vi "ballScrewControl.vi"(0 "joy1Wheel":dbl, 1 "button8":bool, 4 "button7":bool, 5 "ballScrewMotorIN":T1={"DeviceStatus"={"status"=FALSE, "code"=0, "source"=""}, "Type"=enum."PWM", "PWM"={"Digital Module"=enum."Digital Module 2", "PWM Channel"=enum."PWM 1", "DeadBand"={"Name"="", "maxPositivePwm"=0, "minPositivePwm"=0, "centerPwm"=0, "maxNegativePwm"=0, "minNegativePwm"=0, "angularRange"=0}}, "CAN"={"Device Number"=0, "Control Mode"=enum."Percent VBus", "Semaphore"=refnum, "Max Vout"=12.0}, "Invert"=FALSE, "TransformRef"=refnum, "InvTransformRef"=refnum}, 6 "Distance":dbl, 7 "joy2YAxis":dbl, 8 "autoTrackingButton":bool, 9 "closedLoopKillButton":bool, 10 "ballScrewBotLimitSwitch":bool, 11 "ballScrewTopLimitSwitch":bool) -> (2 "motorValueOutput":dbl, 3 "ballScrewMotorOUT":T1={"DeviceStatus"={"status"=FALSE, "code"=0, "source"=""}, "Type"=enum."PWM", "PWM"={"Digital Module"=enum."Digital Module 1", "PWM Channel"=enum."Invalid", "DeadBand"={"Name"="", "maxPositivePwm"=0, "minPositivePwm"=0, "centerPwm"=0, "maxNegativePwm"=0, "minNegativePwm"=0, "angularRange"=0}}, "CAN"={"Device Number"=0, "Control Mode"=enum."Percent VBus", "Semaphore"=refnum, "Max Vout"=12.0}, "Invert"=FALSE, "TransformRef"=refnum, "InvTransformRef"=refnum})   [LabVIEW 2012]
uses:
  <vilib>/Rock Robotics/WPI/MotorControl/WPI_MotorControlDeviceRef.ctl
  <vilib>/Rock Robotics/SystemInterfaces/Typedef/FPGA_TypedefDigitalModule.ctl
  <vilib>/Rock Robotics/SystemInterfaces/DIO/FPGA_DIOPWMChannel.ctl
  <vilib>/Rock Robotics/WPI/PWM/WPI_PWMDeadband.ctl
  <vilib>/Rock Robotics/WPI/CAN/Jaguar/SubVIs/WPI_CANJaguar_ControlMode.ctl
  <vilib>/Rock Robotics/WPI/PWM/WPI_PWMTransform_ConPane.ctl
  <vilib>/Rock Robotics/WPI/CAN/Jaguar/SubVIs/WPI_CANJaguar_StatusSelect.ctl
  <vilib>/Rock Robotics/WPI/CAN/Jaguar/SubVIs/WPI_CANJaguar_StatusChannelSelect.ctl
  <vilib>/Rock Robotics/WPI/DriverStation/DriverStationLCD/WPI_DriverStationLCDLCDLine.ctl
  <vilib>/Rock Robotics/WPI/CAN/Jaguar/SubVIs/WPI_CANJaguar_BrakeCoastMode.ctl
  2013NewCan/Robot Global Data.vi
panel:
  out "POT FEEDBACK":dbl
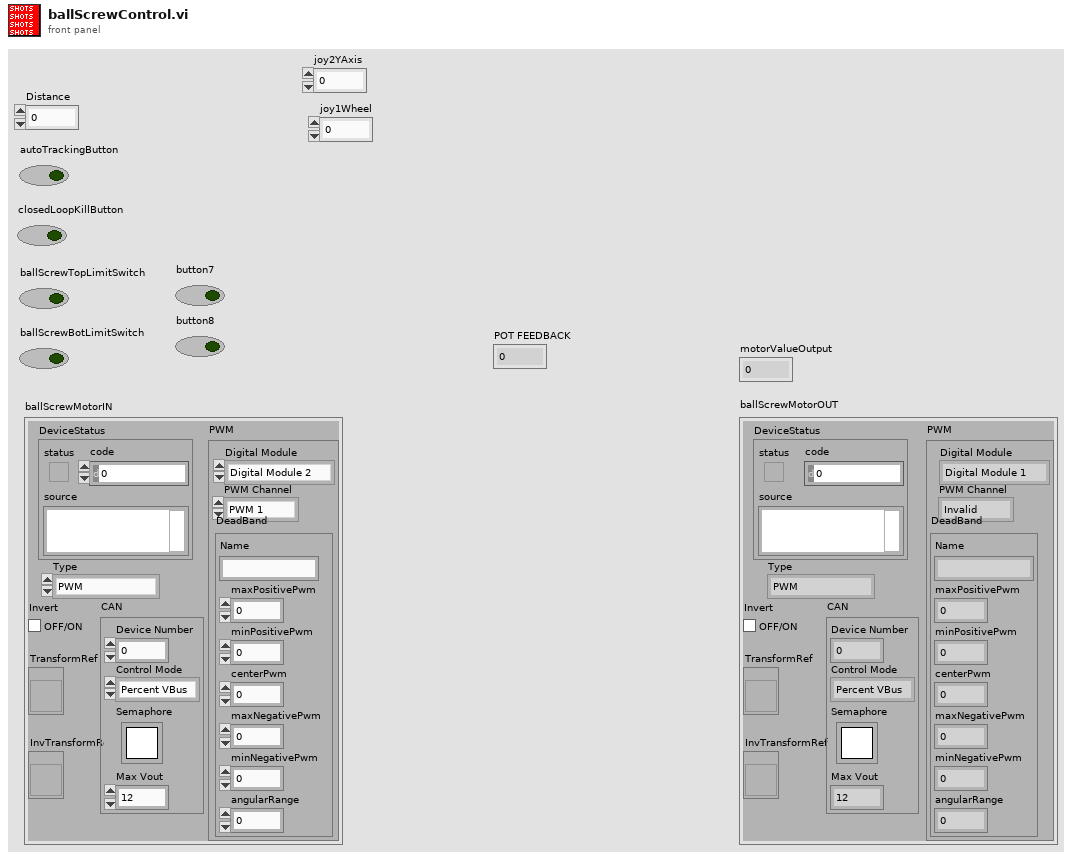
[diagram p1: front panel]
types:
  T1 = typedef "WPI_MotorControlDeviceRef.ctl" = cluster{"DeviceStatus":errorcluster, "Type":enum16{"PWM", "CAN"}, "PWM":cluster{"Digital Module":T2, "PWM Channel":T3, "DeadBand":T4}, "CAN":cluster{"Device Number":u8, "Control Mode":T5, "Semaphore":T6, "Max Vout":dbl}, "Invert":bool, "TransformRef":T7, "InvTransformRef":T7}
  T2 = typedef "FPGA_TypedefDigitalModule.ctl" = enum16{"Digital Module 1", "Digital Module 2"}
  T3 = typedef "FPGA_DIOPWMChannel.ctl" = enum8{"PWM 1", "PWM 2", "PWM 3", "PWM 4", "PWM 5", "PWM 6", "PWM 7", "PWM 8", "PWM 9", "PWM 10", "Invalid"}
  T4 = typedef "WPI_PWMDeadband.ctl" = cluster{"Name":string, "maxPositivePwm":i32, "minPositivePwm":i32, "centerPwm":i32, "maxNegativePwm":i32, "minNegativePwm":i32, "angularRange":u16}
  T5 = typedef "WPI_CANJaguar_ControlMode.ctl" = enum8{"Percent VBus", "Current", "Speed", "Position", "Voltage"}
  T6 = typedef "Semaphore RefNum" = refnum<k1>
  T7 = typedef "WPI_PWMTransform_ConPane.ctl" = refnum<vi>
  T8 = typedef "WPI_DriverStationLCDLCDLine.ctl" = enum16{"Main - Line 1", "User - Line 2", "User - Line 3", "User - Line 4", "User - Line 5", "User - Line 6"}
  T9 = typedef "WPI_CANJaguar_StatusChannelSelect.ctl" = enum16{"Periodic Status Channel 1", "Periodic Status Channel 2", "Periodic Status Channel 3", "Periodic Status Channel 4", "On Demand Status"}
  T10 = typedef "WPI_CANJaguar_StatusSelect.ctl" = enum16{"Output Percent VBus", "Output Voltage", "Bus Voltage", "Current", "Temperature", "Position", "Speed", "Limit Switches", "Faults", "Fault Counters", "Power Cycle"}
  T11 = typedef "WPI_CANJaguar_Status.ctl" = cluster{"Output Percent VBus":dbl, "Output Voltage":dbl, "Bus Voltage":dbl, "Current":dbl, "Temperature":dbl, "Position":dbl, "Speed":dbl, "Limits":cluster{"Forward Limit":bool, "Reverse Limit":bool, "Forward Soft Limit":bool, "Reverse Soft Limit":bool, "Sticky Forward Limit":bool, "Sticky Reverse Limit":bool, "Sticky Forward Soft Limit":bool, "Sticky Reverse Soft Limit":bool}, "Faults":cluster{"Current Fault":bool, "Temperature Fault":bool, "Bus Voltage Fault":bool, "Gate Driver Fault":bool, "Comm Fault":bool}, "Fault Counters":cluster{"Current Faults":u8, "Temperature Faults":u8, "Bus Voltage Faults":u8, "Gate Driver Faults":u8, "Comm Faults":u8, "CAN Status":u8, "CAN RX Errors":u8, "CAN TX Errors":u8}, "Power Cycle":bool}
  T12 = typedef "WPI_CANJaguar_BrakeCoastMode.ctl" = enum8{"Jumper", "Brake", "Coast"}
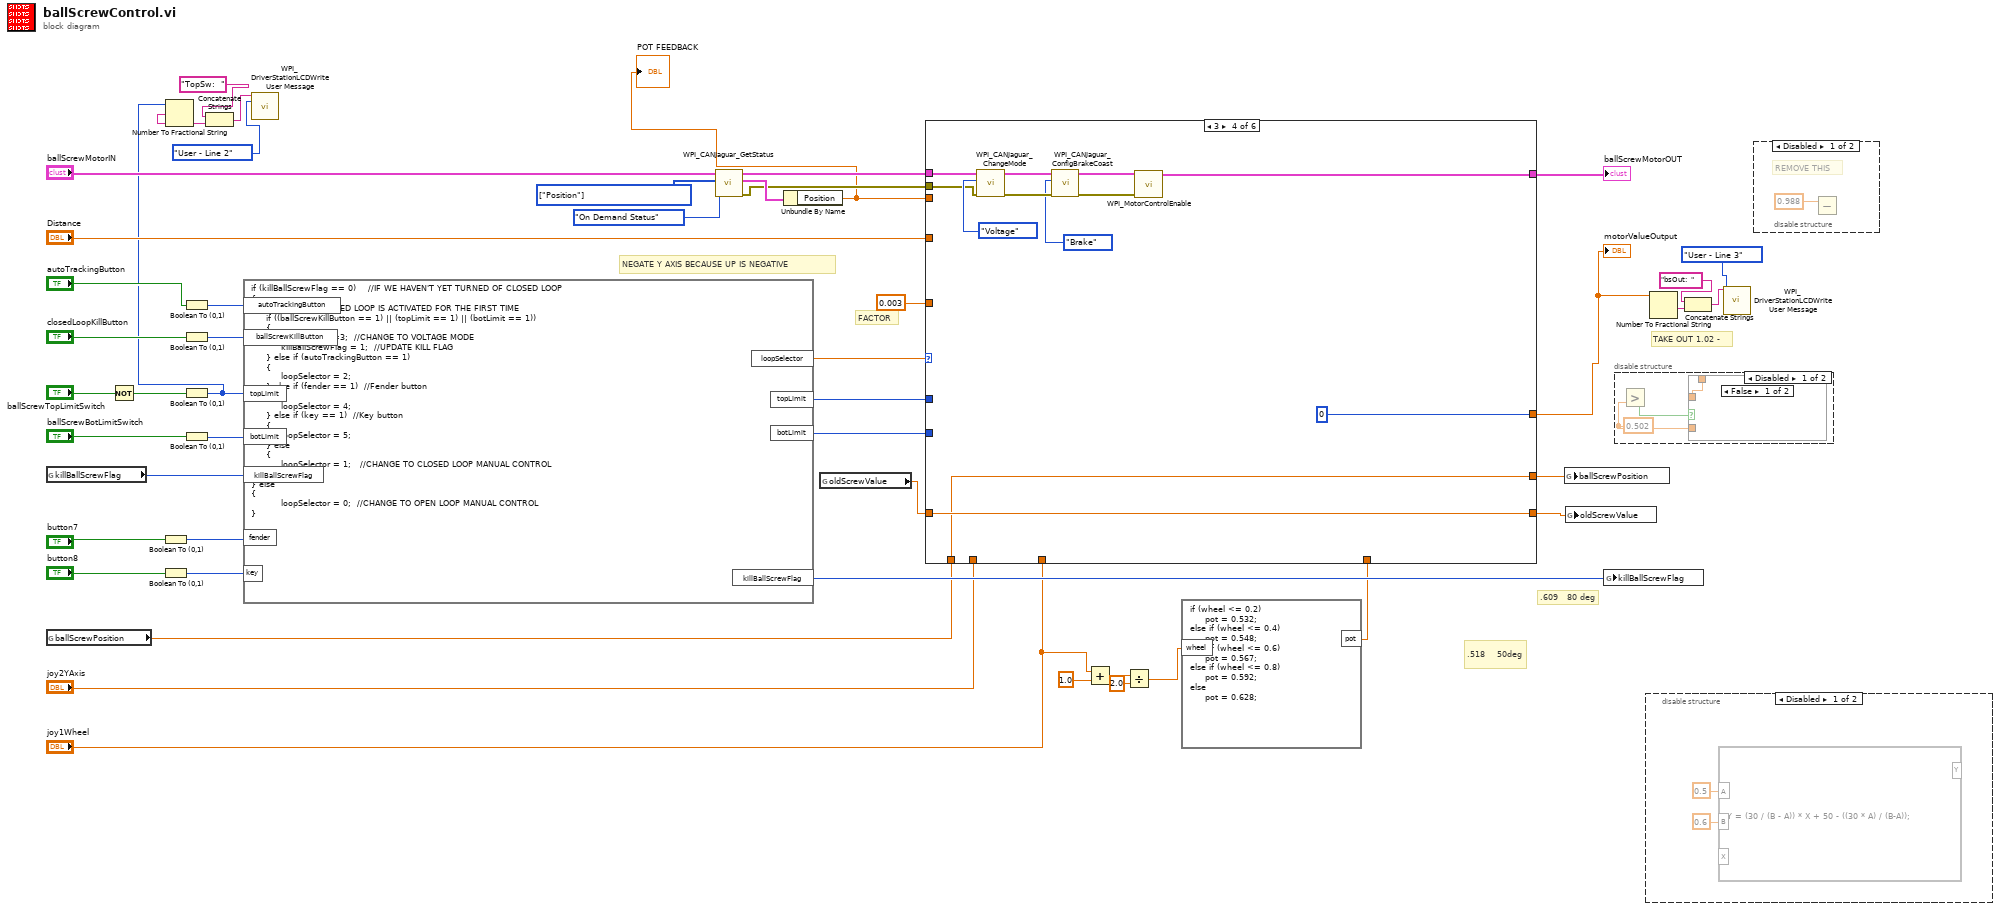
[diagram p0: block diagram]
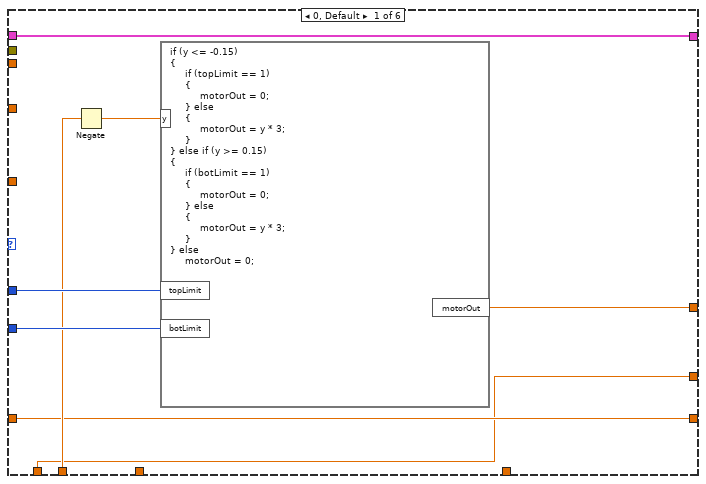
[diagram p6: hidden frame]
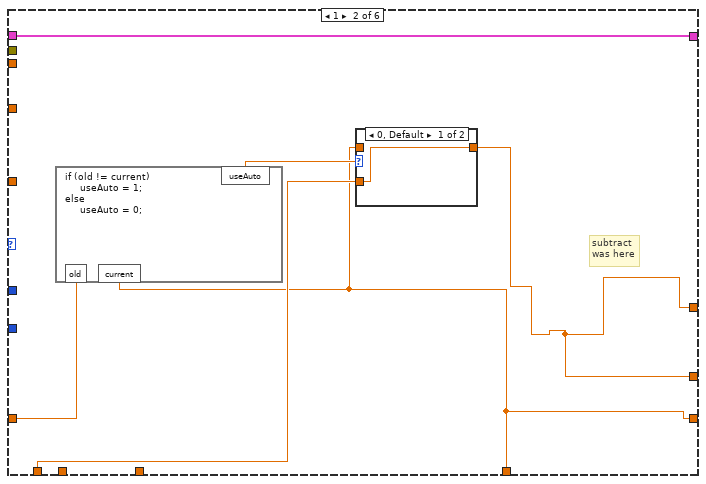
[diagram p7: hidden frame]
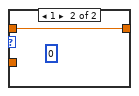
[diagram p8: hidden frame]
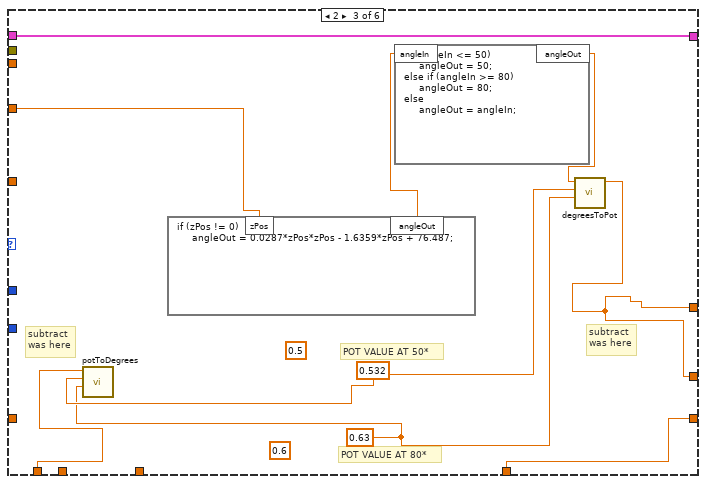
[diagram p9: hidden frame]
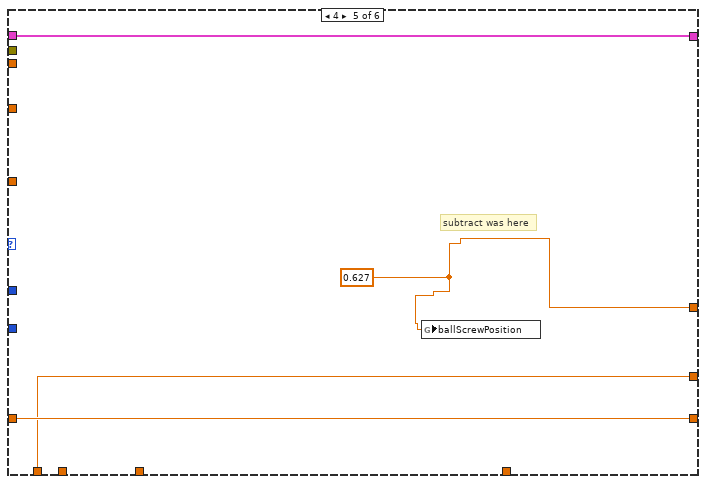
[diagram p10: hidden frame]
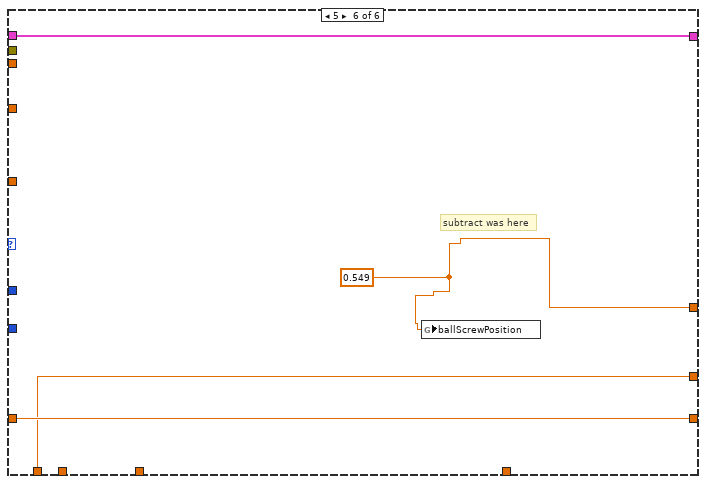
[diagram p11: hidden frame]
diagram:
  w30 = T10[] [enum."Position"] items=["Output Percent VBus", "Output Voltage", "Bus Voltage", "Current", "Temperature", "Position", "Speed", "Limit Switches", "Faults", "Fault Counters", "Power Cycle"] ("Status Select")
  # ".609   80 deg"
  # ".518    50deg"
  # "TAKE OUT 1.02 -"
  # "FACTOR"
  # "NEGATE Y AXIS BECAUSE UP IS NEGATIVE"
  n1 = global read "Robot Global Data.vi" "killBallScrewFlag"() -> (w47:i8)
  n2 = global read "Robot Global Data.vi" "ballScrewPosition"() -> (w34:dbl)
  n3 = Not(x="ballScrewTopLimitSwitch") -> (.not. x?=w32:bool)
  n4 = Boolean To (0,1)(Boolean="button7") -> (0, 1=w18:i16)
  n5 = Boolean To (0,1)(Boolean="button8") -> (0, 1=w2:i16)
  n6 = Boolean To (0,1)(Boolean="autoTrackingButton") -> (0, 1=w36:i16)
  n7 = Boolean To (0,1)(Boolean="closedLoopKillButton") -> (0, 1=w48:i16)
  n8 = Boolean To (0,1)(Boolean=w32) -> (0, 1=w19:i16)
  n9 = Number To Fractional String(number=w19) -> (F-format string=w23:string)  [unwired: 3 in]
  n10 = Boolean To (0,1)(Boolean="ballScrewBotLimitSwitch") -> (0, 1=w24:i16)
  n11 = Concatenate Strings("TopSw:  " ("line text"), w23) -> (w22:string)
  n12 = formula code="if (killBallScrewFlag == 0)    //IF WE HAVEN'T YET TURNED OF CLOSED LOOP\n{\n     //IF THE KILL CLOSED LOOP IS ACTIVATED FOR THE FIRST TIME\n     if ((ballScrewKillButton == 1) || (topLimit == 1) || (botLimit == 1))\n     {\n          loopSelector =3;  //CHANGE TO VOLTAGE MODE\n          killBallScrewFlag = 1;  //UPDATE KILL FLAG\n     } else if (autoTrackingButton == 1)\n     {\n          loopSelector = 2;\n     } else if (fender == 1)  //Fender button\n     {\n          loopSelector = 4;\n     } else if (key == 1)  //Key button\n     {\n          loopSelector = 5;\n     } else\n     {\n          loopSelector = 1;   //CHANGE TO CLOSED LOOP MANUAL CONTROL\n     }\n} else\n{\n          loopSelector = 0;  //CHANGE TO OPEN LOOP MANUAL CONTROL\n}"("ballScrewKillButton"=w48, "killBallScrewFlag"=w47, "botLimit"=w24, "topLimit"=w19, "autoTrackingButton"=w36, "fender"=w18, "key"=w2) -> ("loopSelector"=w25:dbl, "killBallScrewFlag"=w43:i8, "topLimit"=w38:i16, "botLimit"=w39:i16)
  n13 = call <vilib>:"WPI_DriverStationLCDWrite User Message.vi"("line text"=w22, "line"=WPI_DriverStationLCDLCDLine."User - Line 2") -> ()  [unwired: 13 in, 1 out]
  n14 = call <vilib>:"WPI_CANJaguar_GetStatus.vi"("Status Channel Select"=WPI_CANJaguar_StatusChannelSelect."On Demand Status", "Status Select"=w30, "CAN Jaguar Ref"="ballScrewMotorIN") -> ("error out"=w31:errorcluster, "Status"=w40:T11, "CAN Jaguar Ref Out"=w41:T1)  [unwired: 6 in]
  n15 = Unbundle By Name(w40) -> ("Position"=w28:dbl)
  "POT FEEDBACK" <- w28
  n16 = global read "Robot Global Data.vi" "oldScrewValue"() -> (w9:dbl)
  n17 = Add(x="joy1Wheel", y=1.0) -> (x+y=w15:dbl)
  n18 = Divide(x=w15, y=2.0) -> (x/y=w13:dbl)
  n19 = formula code="if (wheel <= 0.2)\n     pot = 0.532;\nelse if (wheel <= 0.4)\n     pot = 0.548;\nelse if (wheel <= 0.6)\n     pot = 0.567;\nelse if (wheel <= 0.8)\n     pot = 0.592;\nelse\n     pot = 0.628;"("wheel"=w13) -> ("pot"=w11:dbl)
  n20 = case shown="3" w25 {
    tunnel: w41 -> [w56 w62 w73 w85 w89 w93]
    tunnel: [w56 w62 w73 w84 w89 w93] -> w44
    tunnel: w28 -> [_ _ _ _ _ _]
    tunnel: w34 -> [w49 w59 w67 w74 w87 w91]
    tunnel: [w53 w57 w68 0 w86 w90] -> w3
    tunnel: w39 -> [w55 _ _ _ _ _]
    tunnel: w38 -> [w54 _ _ _ _ _]
    tunnel: 0.003 ("input variable") -> [_ _ _ _ _ _]
    tunnel: w31 -> [_ _ _ w81 _ _]
    tunnel: "Distance" -> [_ _ w70 _ _ _]
    tunnel: "joy1Wheel" -> [_ _ _ _ _ _]
    tunnel: "joy2YAxis" -> [w51 _ _ _ _ _]
    tunnel: w11 -> [_ w58 w69 _ _ _]
    tunnel: [w50 w58 w69 w75 w88 w92] -> w10
    tunnel: w9 -> [w50 w61 _ w75 w88 w92]
    tunnel: [w49 w57 w68 w74 w87 w91] -> w8
    frame 0, Default {
      n21 = Negate(x=w51) -> (-x=w52:dbl)
      n22 = formula code="if (y <= -0.15)\n{\n     if (topLimit == 1)\n     {\n          motorOut = 0;\n     } else\n     {\n          motorOut = y * 3;\n     }\n} else if (y >= 0.15)\n{\n     if (botLimit == 1)\n     {\n          motorOut = 0;\n     } else\n     {\n          motorOut = y * 3;\n     }\n} else\n     motorOut = 0;"("topLimit"=w54, "botLimit"=w55, "y"=w52) -> ("motorOut"=w53:dbl)
    }
    frame 1 {
      # "subtract\nwas here"
      n23 = formula code="if (old != current)\n     useAuto = 1;\nelse\n     useAuto = 0;"("old"=w61, "current"=w58) -> ("useAuto"=w60:dbl)
      n24 = case shown="0, Default" w60 {
        tunnel: [w63 w64] -> w57
        tunnel: w58 -> [_ w64]
        tunnel: w59 -> [w63 _]
        frame 0, Default {
        }
        frame 1 {
          (unwired) 0
        }
      }
    }
    frame 2 {
      (unwired) 0.6
      (unwired) 0.5
      w71 = 0.63
      w72 = 0.532
      # "subtract\nwas here"
      # "subtract\nwas here"
      # "POT VALUE AT 50*"
      # "POT VALUE AT 80*"
      n25 = call "potToDegrees.vi"("POT VALUE AT 80*"=w71, "POT VALUE AT 50*"=w72, "POT VALUE"=w67) -> ()  [unwired: 8 in, 1 out]
      n26 = formula code="if (zPos != 0)\n     angleOut = 0.0287*zPos*zPos - 1.6359*zPos + 76.487;"("zPos"=w70) -> ("angleOut"=w66:dbl)
      n27 = formula code="if (angleIn <= 50)\n     angleOut = 50;\nelse if (angleIn >= 80)\n     angleOut = 80;\nelse\n     angleOut = angleIn;"("angleIn"=w66) -> ("angleOut"=w65:dbl)
      n28 = call "degreesToPot.vi"("POT VALUE AT 80*"=w71, "POT VALUE AT 50*"=w72, "ANGLE(DEGREES)"=w65) -> ("POT VALUE (0-1)"=w68:dbl)  [unwired: 8 in]
    }
    frame 3 {
      n29 = call <vilib>:"WPI_CANJaguar_ChangeMode.vi"("error in (no error)"=w81, "Control Mode"=WPI_CANJaguar_ControlMode."Voltage", "CAN Jaguar Ref"=w85) -> ("error out"=w79:errorcluster, "CAN Jaguar Ref Out"=w80:T1)  [unwired: 7 in]
      n30 = call <vilib>:"WPI_CANJaguar_ConfigBrakeCoast.vi"("error in (no error)"=w79, "Brake / Coast Mode"=WPI_CANJaguar_BrakeCoastMode."Brake", "CAN Jaguar Ref"=w80) -> ("error out"=w78:errorcluster, "CAN Jaguar Ref Out"=w77:T1)  [unwired: 7 in]
      n31 = call <vilib>:"WPI_MotorControlEnable.vi"("error in (no error)"=w78, "CAN Jaguar Ref"=w77) -> ("CAN Jaguar Ref Out"=w84:T1)  [unwired: 8 in, 1 out]
    }
    frame 4 {
      w86 = 0.627 ("ballScrewPosition")
      # "subtract was here"
      n32 = global write "Robot Global Data.vi" "ballScrewPosition"(w86) -> ()
    }
    frame 5 {
      w90 = 0.549 ("ballScrewPosition")
      # "subtract was here"
      n33 = global write "Robot Global Data.vi" "ballScrewPosition"(w90) -> ()
    }
  }
  "ballScrewMotorOUT" <- w44
  "motorValueOutput" <- w3
  n34 = global write "Robot Global Data.vi" "ballScrewPosition"(w8) -> ()
  n35 = global write "Robot Global Data.vi" "oldScrewValue"(w10) -> ()
  n36 = global write "Robot Global Data.vi" "killBallScrewFlag"(w43) -> ()
  n37 = disable-structure shown="Disabled" {
    frame Disabled {
      w94 = 0.502 ("y")
      n38 = Greater?(y=w94) -> (0:w95:bool)  [unwired: 1 in]
      n39 = case shown="False" w95 {
        tunnel: [w96 w97] -> _
        tunnel: _ -> [w96 _]
        tunnel: w94 -> [_ w97]
        frame False {
        }
        frame True {
        }
      }
    }
    frame Enabled {
    }
  }
  n40 = disable-structure shown="Disabled" {
    frame Disabled {
      n41 = formula code="Y = (30 / (B - A)) * X + 50 - ((30 * A) / (B-A));"("B"=0.6 ("input variable"), "A"=0.5 ("input variable")) -> ("X"=w98:dbl)  [unwired: 1 out]
    }
    frame Enabled {
    }
  }
  n42 = Number To Fractional String(number=w3) -> (F-format string=w4:string)  [unwired: 3 in]
  n43 = Concatenate Strings("bsOut:  " ("line text"), w4) -> (w5:string)
  n44 = call <vilib>:"WPI_DriverStationLCDWrite User Message.vi"("line text"=w5, "line"=WPI_DriverStationLCDLCDLine."User - Line 3") -> ()  [unwired: 13 in, 1 out]
  n45 = disable-structure shown="Disabled" {
    frame Disabled {
      # "REMOVE THIS"
      n46 = Subtract(x=0.988) -> ()  [unwired: 1 in, 1 out]
    }
    frame Enabled {
    }
  }
